vi "CD Engine lvlib.vi"(9 "Action":T1) -> (1 "Output":string)   [LabVIEW 2019, in "NIVS_Consolidated_CDW_MetaDataObj.lvclass"]
doc: "Constants, which are necessary for the <B>CD Engine library</B> in the generated custom device project."
uses:
  NIVS_Consolidated_CDW_MetaDataObj.lvclass
  CD Engine lvlib.ctl
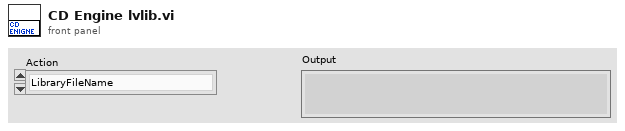
[diagram p1: front panel]
types:
  T1 = typedef "NIVS_Consolidated_CDW_MetaDataObj.lvclass/CD Engine lvlib.ctl" = enum16{"LibraryFileName", "LibraryFolderName", "Engine.FolderName", "Engine.Init.FolderName", "Engine.Run.FolderName", "Engine.Shutdown.FolderName", "Types.FolderName", "Engine.RT Driver VI.TemplatePath", "Engine.RT Driver VI.FileName", "Engine.PPL.RT Driver VI_InlineAsync.FileName", "Engine.RTStateVariables.Name", "Engine.PPL.RTStateVariables.Name", "Engine.RTStateVariables.Name.NoExtension", "Engine.Async.NameExtension", "Engine.Async.TemplateName", "Engine.PPL.Async.TemplateName", "Engine.PPL.Async.InitVSGlobals.Name", "Engine.PPL.RT Driver VI_Inline.FileName"}
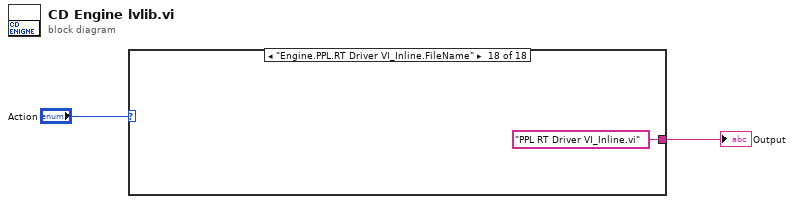
[diagram p0: block diagram]
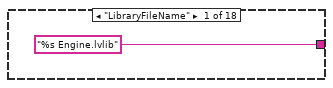
[diagram p2: hidden frame]
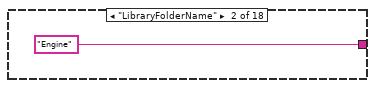
[diagram p3: hidden frame]
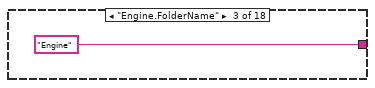
[diagram p4: hidden frame]
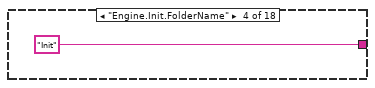
[diagram p5: hidden frame]
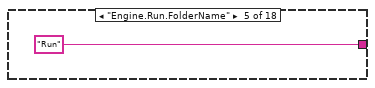
[diagram p6: hidden frame]
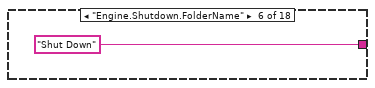
[diagram p7: hidden frame]
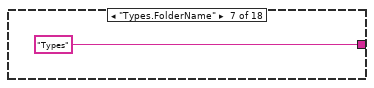
[diagram p8: hidden frame]
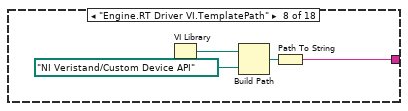
[diagram p9: hidden frame]
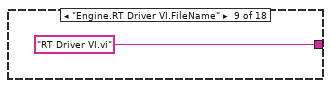
[diagram p10: hidden frame]
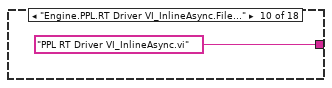
[diagram p11: hidden frame]
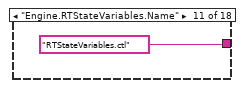
[diagram p12: hidden frame]
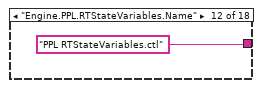
[diagram p13: hidden frame]
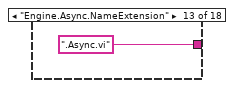
[diagram p14: hidden frame]
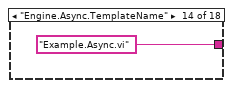
[diagram p15: hidden frame]
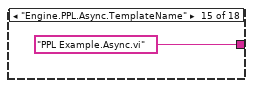
[diagram p16: hidden frame]
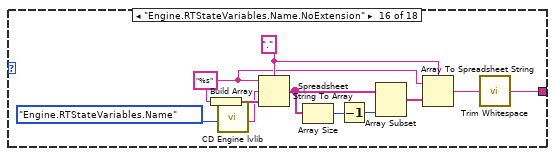
[diagram p17: hidden frame]
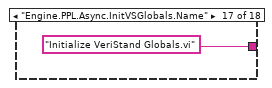
[diagram p18: hidden frame]
diagram:
  n1 = case shown="\"Engine.PPL.RT Driver VI_Inline.FileName\"" "Action" {
    tunnel: ["%s Engine.lvlib" "Engine" "Engine" "Init" "Run" "Shut Down" "Types" w10 "RT Driver VI.vi" "PPL RT Driver VI_InlineAsync.vi" "RTStateVariables.ctl" ("Output") "PPL RTStateVariables.ctl" ("Output") ".Async.vi" ("name or relative path") "Example.Async.vi" ("name or relative path") "PPL Example.Async.vi" ("name or relative path") w21 "Initialize VeriStand Globals.vi" ("trimmed string") "PPL RT Driver VI_Inline.vi" ("trimmed string")] -> w1
    frame "LibraryFileName" {
    }
    frame "LibraryFolderName" {
    }
    frame "Engine.FolderName" {
    }
    frame "Engine.Init.FolderName" {
    }
    frame "Engine.Run.FolderName" {
    }
    frame "Engine.Shutdown.FolderName" {
    }
    frame "Types.FolderName" {
    }
    frame "Engine.RT Driver VI.TemplatePath" {
      n2 = VI Library() -> (path=w11:path)
      n3 = Build Path(base path=w11, name or relative path=path "NI Veristand/Custom Device API") -> (appended path=w13:path)
      n4 = Path To String(path=w13) -> (string=w10:string)
    }
    frame "Engine.RT Driver VI.FileName" {
    }
    frame "Engine.PPL.RT Driver VI_InlineAsync.FileName" {
    }
    frame "Engine.RTStateVariables.Name" {
    }
    frame "Engine.PPL.RTStateVariables.Name" {
    }
    frame "Engine.Async.NameExtension" {
    }
    frame "Engine.Async.TemplateName" {
    }
    frame "Engine.PPL.Async.TemplateName" {
    }
    frame "Engine.RTStateVariables.Name.NoExtension" {
      w26 = "." ("delimiter (Tab)")
      w25 = "%s" ("format string")
      n5 = Build Array(w25) -> (w31:string[])
      n6 = call "CD Engine lvlib.vi"("Action"=CD_Engine_lvlib."Engine.RTStateVariables.Name") -> ("Output"=w23:string)  [unwired: 10 in]
      n7 = Spreadsheet String To Array(delimiter (Tab)=w26, format string=w25, spreadsheet string=w23, array type (2D Dbl)=w31) -> (array=w30:string[])
      n8 = Array Size(array=w30) -> (size(s)=w29:i32)
      n9 = Decrement(x=w29) -> (x-1=w28:i32)
      n10 = Array Subset(array=w30, length=w28) -> (w27:string[])  [unwired: 1 in]
      n11 = Array To Spreadsheet String(delimiter (Tab)=w26, array=w27, 3:w25) -> (spreadsheet string=w22:string)
      n12 = call <vilib>:"Trim Whitespace.vi"("string"=w22) -> ("trimmed string"=w21:string)  [unwired: 1 in]
    }
    frame "Engine.PPL.Async.InitVSGlobals.Name" {
    }
    frame "Engine.PPL.RT Driver VI_Inline.FileName" {
    }
  }
  "Output" <- w1
